vi "pasu.vi"() -> ()   [LabVIEW 2013]
uses:
  <vilib>/Analysis/NI_AALBase.lvlib
  <vilib>/Analysis/baseanly.llb/Mean (DBL).vi
panel:
  in  "Запуск системы:":bool
  in  "Код кнфигурации":i16
  in  "Канал ЦАП:":i16
  in  "Код конфигурации:":i16
  in  "Код конфигурации:":i16
  out "Напряжение на фоторезисторе, В":dbl
  in  "Канал АЦП шунта:":i16
  out "Ток в цепи освещения, А":dbl
  out "Состояние системы:":bool
  in  "Частота регистрации данных, с:":i16
  in  "Путь к log файлу:":path
  in  "Канал АЦП фоторезистора:":i16
  in  "Порог срабатывания подсветки, В":dbl
  out "Дата и время срабатывания:":string
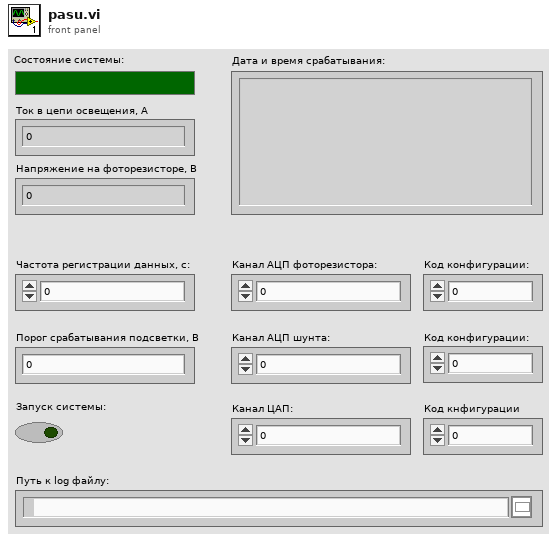
[diagram p1: front panel]
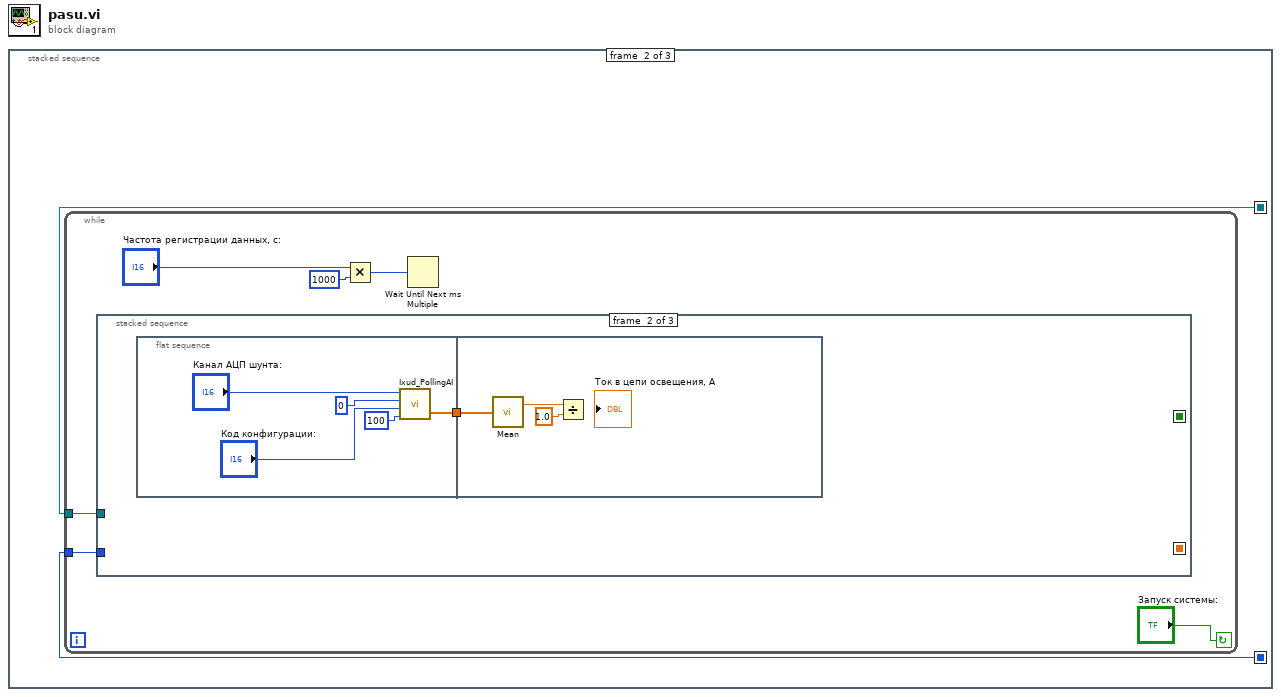
[diagram p0: block diagram]
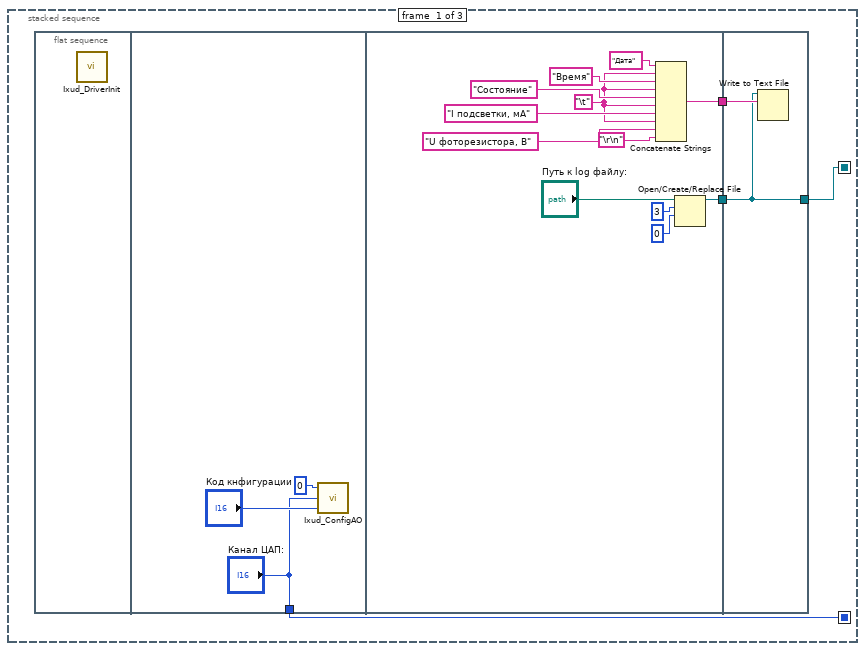
[diagram p2: hidden frame]
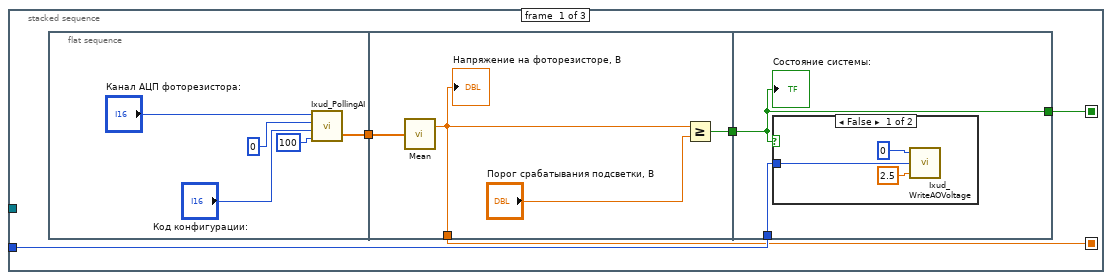
[diagram p3: hidden frame]
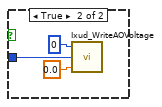
[diagram p4: hidden frame]
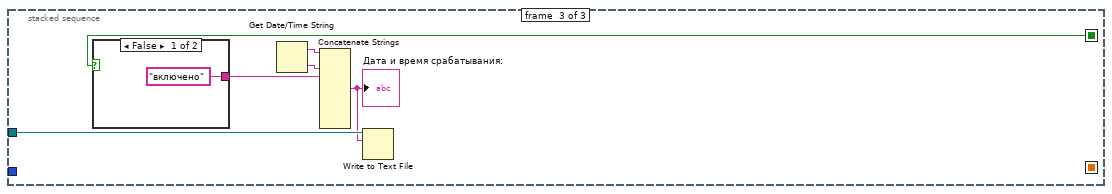
[diagram p5: hidden frame]
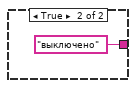
[diagram p6: hidden frame]
diagram:
  n1 = stacked-sequence {
    seq-local: [w2 _ _] -> [_ w23 _]
    seq-local: [w1 _ _] -> [_ w22 _]
    frame #0 {
      n2 = flat-sequence {
        tunnel: ["Канал ЦАП:"] -> w2
        tunnel: [w9] -> w4
        tunnel: [w8] -> w3
        tunnel: w4 -> [w20]
        tunnel: w3 -> [w21]
        tunnel: [w20] -> w1
        frame #0 {
          n3 = call "Ixud_DriverInit.vi"() -> ()  [unwired: 2 out]
        }
        frame #1 {
          n4 = call "Ixud_ConfigAO.vi"("wCfgCode"="Код кнфигурации", "wChannel"="Канал ЦАП:", "wBoardNo"=0) -> ()  [unwired: 1 out]
        }
        frame #2 {
          w11 = "\t"
          n5 = Concatenate Strings("Дата", w11, "Время", w11, "Состояние", w11, "I подсветки, мА", w11, "U фоторезистора, В", "\r\n") -> (w8:string)
          n6 = Open/Create/Replace File(file path (use dialog)="Путь к log файлу:", operation (0:open)=3, access (0:read/write)=0) -> (refnum out=w9:refnum<file>)  [unwired: 3 in, 2 out]
        }
        frame #3 {
          n7 = Write to Text File(file (use dialog)=w20, text=w21) -> ()  [unwired: 2 in, 3 out]
        }
      }
    }
    frame #1 {
      n8 = while {
        tunnel: w23 -> [w25]
        tunnel: w22 -> [w24]
        stop <- "Запуск системы:" continue-if-true
        n9 = stacked-sequence {
          seq-local: [w31 _ _] -> [_ _ w64]
          seq-local: [w30 _ _] -> [_ _ _]
          tunnel: w25 -> [w32 _ _]
          tunnel: w24 -> [_ _ w62]
          frame #0 {
            n10 = flat-sequence {
              tunnel: [w35] -> w34
              tunnel: w34 -> [w43]
              tunnel: [w41] -> w30
              tunnel: [w40] -> w33
              tunnel: w33 -> [w44]
              tunnel: w32 -> [w45]
              tunnel: [w44] -> w31
              frame #0 {
                n11 = call "Ixud_PollingAI.vi"("dwDataCount"=100, "wConfig"="Код конфигурации:", "wBoardNo"=0, "wChannel"="Канал АЦП фоторезистора:") -> ("fValue"=w35:sgl[])  [unwired: 1 out]
              }
              frame #1 {
                n12 = call-poly <vilib>:"Mean.vi"("X"=w43) -> ("mean"=w41:dbl)  [unwired: 1 out]
                "Напряжение на фоторезисторе, В" <- w41
                n13 = Greater Or Equal?(x=w41, y="Порог срабатывания подсветки, В") -> (x >= y?=w40:bool)
              }
              frame #2 {
                n14 = case shown="False" w44 {
                  tunnel: w45 -> [w47 w51]
                  frame False {
                    n15 = call "Ixud_WriteAOVoltage.vi"("fValue"=sgl 2.5, "wChannel"=w47, "wBoardNo"=u16 0) -> ()  [unwired: 1 out]
                  }
                  frame True {
                    n16 = call "Ixud_WriteAOVoltage.vi"("fValue"=sgl 0.0, "wChannel"=w51, "wBoardNo"=u16 0) -> ()  [unwired: 1 out]
                  }
                }
                "Состояние системы:" <- w44
              }
            }
          }
          frame #1 {
            n17 = flat-sequence {
              tunnel: [w53] -> w52
              tunnel: w52 -> [w60]
              frame #0 {
                n18 = call "Ixud_PollingAI.vi"("dwDataCount"=u32 100, "wConfig"="Код конфигурации:", "wBoardNo"=0, "wChannel"="Канал АЦП шунта:") -> ("fValue"=w53:sgl[])  [unwired: 1 out]
              }
              frame #1 {
                n19 = call-poly <vilib>:"Mean.vi"("X"=w60) -> ("mean"=w58:dbl)  [unwired: 1 out]
                n20 = Divide(x=w58, y=1.0) -> ()  [unwired: 1 out]
              }
            }
          }
          frame #2 {
            n21 = case shown="False" w64 {
              tunnel: ["включено" "выключено"] -> w63
              frame False {
              }
              frame True {
              }
            }
            n22 = Get Date/Time String() -> (date string=w66:string, time string=w65:string)  [unwired: 3 in]
            n23 = Concatenate Strings(w66, w65, w63) -> (w61:string)  [unwired: 7 in]
            "Дата и время срабатывания:" <- w61
            n24 = Write to Text File(file (use dialog)=w62, text=w61) -> ()  [unwired: 2 in, 3 out]
          }
        }
        n25 = Multiply(x="Частота регистрации данных, с:", y=1000) -> (x*y=w26:i32)
        n26 = Wait Until Next ms Multiple(millisecond multiple=w26) -> ()  [unwired: 1 out]
      }
    }
    frame #2 {
    }
  }
